vi "_API_BINANCE_GET_Price.vi"(0 "BinanceAPI in":refnum<class "BinanceAPI_.lvclass">, 5 "price":cluster{"symbol (BTCUSDT)":string}, 11 "error in (no error)":errorcluster) -> (4 "BinanceAPI out":refnum<class "BinanceAPI_.lvclass">, 6 "lastPrice":dbl format="%#.6g", 14 "Body":string, 15 "error out":errorcluster)   [LabVIEW 2022 SP3, in "BinanceAPI_.lvclass"]
doc: "https://binance-docs.github.io/apidocs/spot/en/#symbol-price-ticker"
uses:
  BinanceAPI_.lvclass
  BinanceAPI_.lvclass/BinanceAPI_.ctl
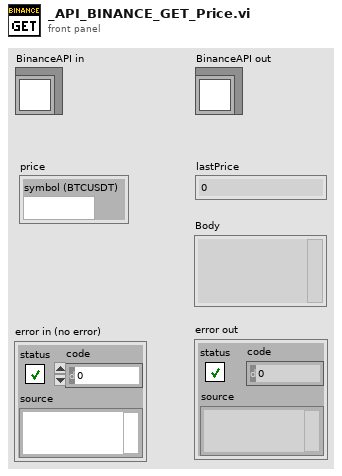
[diagram p1: front panel]
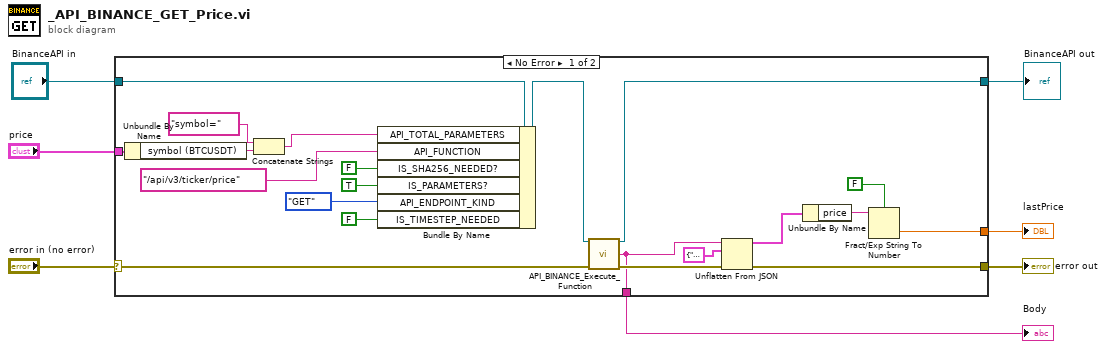
[diagram p0: block diagram]
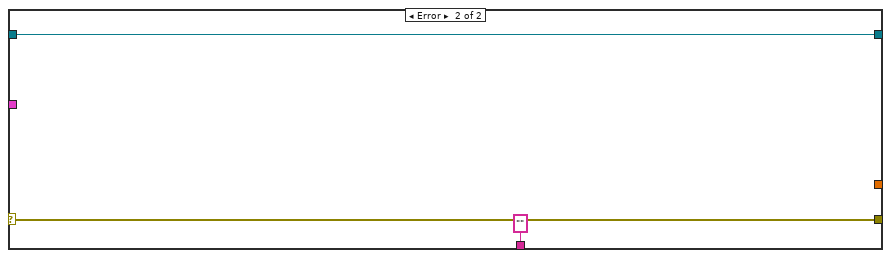
[diagram p2: hidden frame]
diagram:
  n1 = case shown="No Error" "error in (no error)" {
    selector: "error in (no error)" -> [w15 w31]
    tunnel: [w13 w31] -> w5
    tunnel: [w16 w30] -> w1
    tunnel: "BinanceAPI in" -> [w28 w30]
    tunnel: "price" -> [w21 _]
    tunnel: [w11 "" ("Body")] -> w4
    tunnel: [w8 _] -> w3
    frame No Error {
      n2 = Unbundle By Name(w21) -> ("symbol (BTCUSDT)"=w20:string)
      n3 = Concatenate Strings("symbol=", w20) -> (w22:string)
      n4 = Bundle By Name(cluster=w28, "API_TOTAL_PARAMETERS"=w22, "API_FUNCTION"="/api/v3/ticker/price", "IS_SHA256_NEEDED?"=FALSE, "IS_PARAMETERS?"=TRUE, "API_ENDPOINT_KIND"=enum16{"POST", "DELETE", "GET", "PUT"}."GET", "IS_TIMESTEP_NEEDED"=FALSE) -> (w17:refnum<class "BinanceAPI_.lvclass">)
      n5 = call "API_BINANCE_Execute_Function.vi"("BinanceAPI in"=w17, "error in (no error)"=w15) -> ("BinanceAPI out"=w16:refnum<class "BinanceAPI_.lvclass">, "Body"=w11:string, "error out"=w14:errorcluster)  [unwired: 9 in, 2 out]
      n6 = Unflatten From JSON(JSON string=w11, type and defaults=cluster{"symbol":string, "price":string} {"symbol"="", "price"=""}, error in (no error)=w14) -> (value=w12:cluster{"symbol":string, "price":string}, error out=w13:errorcluster)  [unwired: 4 in]
      n7 = Unbundle By Name(w12) -> ("price"=w10:string)
      n8 = Fract/Exp String To Number(use system decimal point (T)=FALSE, string=w10) -> (number=w8:dbl)  [unwired: 2 in, 1 out]
    }
    frame Error {
    }
  }
  "error out" <- w5
  "Body" <- w4
  "lastPrice" <- w3
  "BinanceAPI out" <- w1
